vi "Write Roles.vi"(8 "error in (no error)":errorcluster, 10 "Roles":refnum<class "Role_v2.lvclass">[](array[class]), 11 "Play_v2 in":refnum<class "Play_v2.lvclass">) -> (0 "error out":errorcluster, 3 "Play_v2 out":refnum<class "Play_v2.lvclass">)   [LabVIEW 2023, in "Play_v2.lvclass"]
uses:
  Play_v2.lvclass
  NewRoles/Role_v2_class/Role_v2.lvclass
  Play_v2.lvclass/Play_v2.ctl
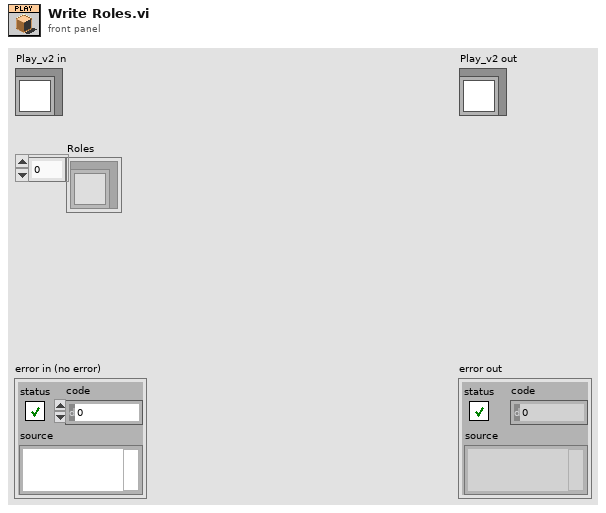
[diagram p1: front panel]
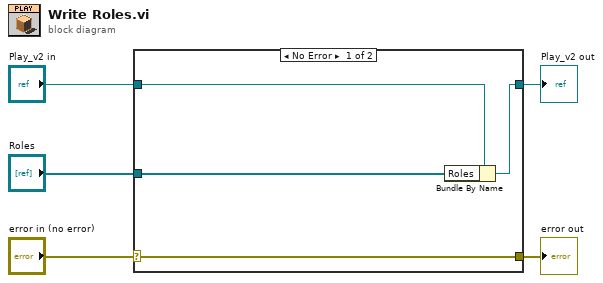
[diagram p0: block diagram]
diagram:
  n1 = case shown="No Error" "error in (no error)" {
    selector: "error in (no error)" -> [w9 w10]
    tunnel: [w9 w10] -> w4
    tunnel: [w7 w11] -> w2
    tunnel: "Play_v2 in" -> [w8 w11]
    tunnel: "Roles" -> [w6 _]
    frame No Error {
      n2 = Bundle By Name(cluster=w8, "Roles"=w6) -> (w7:refnum<class "Play_v2.lvclass">)
    }
    frame Error {
    }
  }
  "error out" <- w4
  "Play_v2 out" <- w2
